vi "Read Time.vi"(11 "Base Teller in":refnum<class "Base Teller.lvclass">) -> (2 "Time":timestamp)   [LabVIEW 2025, in "jettl.lvlib" / "Teller.lvlib" / "Base Teller.lvclass"]
uses:
  Base Teller.lvclass
  Base Teller.lvclass/Base Teller.ctl
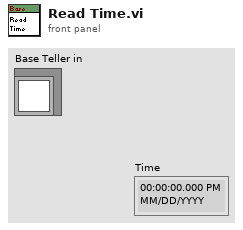
[diagram p1: front panel]
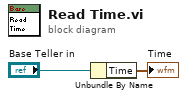
[diagram p0: block diagram]
diagram:
  n1 = Unbundle By Name("Base Teller in") -> ("Time"=→"Time":timestamp)
